vi "CSM - Restore Variable Value.vi"(8 "error in (no error)":errorcluster) -> (2 "error out":errorcluster)   [LabVIEW 2017, in "INI-Static-Variable-Support.lvlib"]
uses:
  INI-Static-Variable-Support.lvlib
  _Support/_fgv-oper.ctl
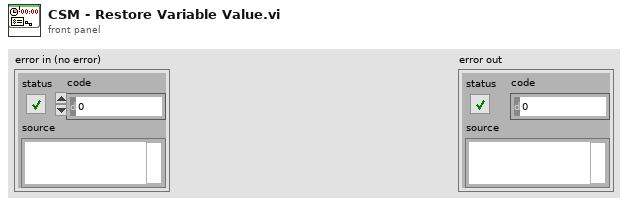
[diagram p1: front panel]
types:
  T1 = typedef "INI-Static-Variable-Support.lvlib/_fgv-oper.ctl" = enum16{"Read", "Write", "Sync", "Sessions", "List Keys", "Load", "List Files", "List Variables", "List Permanent Variables", "Mark Temp Variable as Permenent", "unload", "INIConfig(Memory)", "Reset", "Restore Variable Value"}
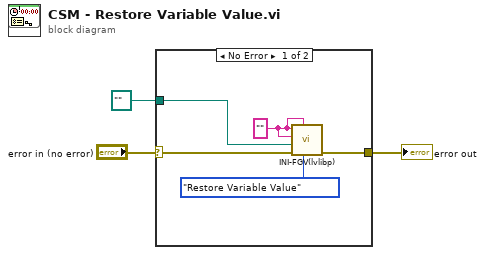
[diagram p0: block diagram]
diagram:
  n1 = case shown="No Error" "error in (no error)" {
    selector: "error in (no error)" -> [w6 w9]
    tunnel: path "" ("Path") -> [w7 _]
    tunnel: [w5 w9] -> w1
    frame No Error {
      w4 = "" (">> Variable Name >>")
      n2 = call "INI-FGV(lvlibp).vi"("Enum"=_fgv-oper."Restore Variable Value", "Prefered Section"=w4, "error IN"=w6, "Path"=w7, ">> Default Value >>"=w4, ">> Variable Name >>"=w4) -> ("error out"=w5:errorcluster)  [unwired: 2 in, 3 out]
    }
    frame Error {
    }
  }
  "error out" <- w1
